vi "Write Session.TCPIP.ConnectTimeout.vi"(8 "error in (no error)":errorcluster, 10 "Session.TCPIP.ConnectTimeout":dbl, 11 "SLSC Remote in":refnum<class "SLSC Remote.lvclass">) -> (0 "error out":errorcluster, 3 "SLSC Remote out":refnum<class "SLSC Remote.lvclass">)   [LabVIEW 2016, in "SLSC Interfaces.lvlib" / "SLSC Remote.lvclass"]
uses:
  SLSC Remote.lvclass
  <vilib>/NI/JSON Support for LabVIEW/JSON Data Classes/JSON Helper/JSON Helper.lvclass
  <vilib>/NI/JSON Support for LabVIEW/JSON Data Classes/JSON Numeric/New JSON Numeric.vi
  <vilib>/NI/JSON Support for LabVIEW/JSON Data Classes/JSON Numeric/JSON Numeric.lvclass
  C:/Program Files (x86)/National Instruments/LabVIEW 2016/vi.lib/National Instruments/JSON Support for LabVIEW/JSON Data Classes/JSON Datatype/JSON Null.lvclass
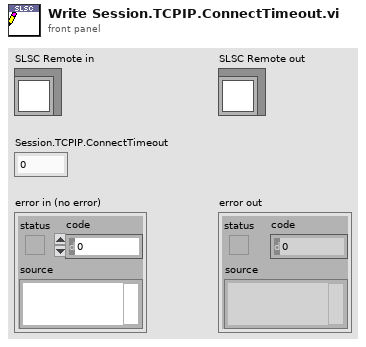
[diagram p1: front panel]
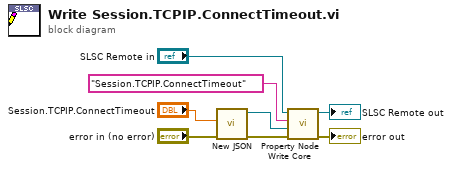
[diagram p0: block diagram]
diagram:
  n1 = call-poly <vilib>:"New JSON.vi"("error in (no error)"="error in (no error)", "value"="Session.TCPIP.ConnectTimeout") -> ("error out"=w4:errorcluster, "JSON String out"=w3:refnum<class "JSON Numeric.lvclass">)  [unwired: 8 in]
  n2 = call "Property Node Write Core.vi"("error in (no error)"=w4, "value"=w3, "property"="Session.TCPIP.ConnectTimeout", "SLSC Remote in"="SLSC Remote in") -> ("error out"=→"error out":errorcluster, "SLSC Remote out"=→"SLSC Remote out":refnum<class "SLSC Remote.lvclass">)  [unwired: 6 in]
